vi "APS motion io status.vi"(0 "Axis_ID":i32, 4 "字符串":string, 5 "error in (no error)":errorcluster caption="错误输入（无错误）") -> (14 "function return":i32, 18 "元素":bool, 19 "error out":errorcluster caption="错误输出")   [LabVIEW 2012, in "APS168.lvlib"]
doc: "I32 FNTYPE APS_motion_io_status( I32 Axis_ID );"
uses:
  APS168.lvlib
  APS168.dll
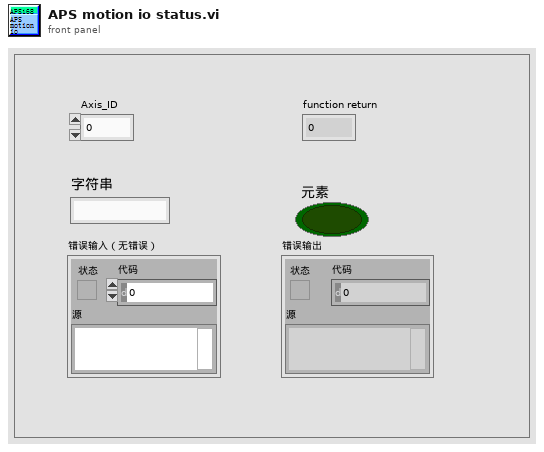
[diagram p1: front panel]
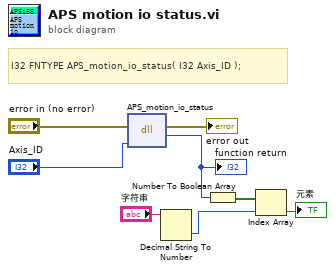
[diagram p0: block diagram]
diagram:
  # "I32 FNTYPE APS_motion_io_status( I32 Axis_ID );"
  n1 = dll-call lib="PTH1,abs E\t冲压机运动204c\nAPS168.dll" fn="APS_motion_io_status"(error in="error in (no error)", "Axis_ID"="Axis_ID") -> (error out=→"error out":errorcluster, "返回类型"=w4:i32)  [unwired: 3 in, 1 out]
  "function return" <- w4
  n2 = Decimal String To Number(string="字符串") -> (number=w2:i32)  [unwired: 2 in, 1 out]
  n3 = Number To Boolean Array(number=w4) -> (Boolean array=w5:bool[])
  n4 = Index Array(array=w5, index=w2) -> (element=→"元素":bool)
